vi "test-quintic-spline-05.vi"() -> ()   [LabVIEW 2019]
uses:
  <vilib>/Rock Robotics/WPI/ThirdParty/JAS_Junk/TrajLib/POSEwCURVATURE.ctl
  <vilib>/Rock Robotics/WPI/ThirdParty/JAS_Junk/TrajLib/POSE2D.ctl
  <vilib>/Rock Robotics/WPI/ThirdParty/JAS_Junk/TrajLib/TRANSLATION2D.ctl
  <vilib>/Rock Robotics/WPI/ThirdParty/JAS_Junk/TrajLib/ROTATION2D.ctl
  <vilib>/Rock Robotics/WPI/ThirdParty/JAS_Junk/TrajLib/Rotation_CreateAngle.vi
  <vilib>/Rock Robotics/WPI/ThirdParty/JAS_Junk/TrajLib/Translation_Create.vi
  <vilib>/Rock Robotics/WPI/ThirdParty/JAS_Junk/TrajLib/Util_CalcDist.vi
  <vilib>/Rock Robotics/WPI/ThirdParty/JAS_Junk/TrajLib/Trajectory_Library.lvlib
panel:
  out "XY Graph":cluster{dbl[], dbl[]}(graph)
  out "Numb\nWaypoints":i32
  out "All Interior \nwayPoints\nFound (True)":bool
  out "end rot = 0":dbl
  out "end y = 0":dbl
  out "end x = 0":dbl
  out "start rot = 0":dbl
  out "start y = 0":dbl
  out "start x = 0":dbl
  out "max dtheta < 0.0872":dbl
  out "max dy < 0.00127":dbl
  out "max dx  < 0.127":dbl
  out "Overall Error":errorcluster
  out "Elements":i32
  out "Create Spline Error":errorcluster
  out "SplinePoses\nWCurve":T1[](array[typedef]) {"POSE"."ROTATION"."SIN" format="%13.4f"; "POSE"."ROTATION"."COS" format="%13.4f"; "POSE"."ROTATION"."VALUE" format="%13.4f"; "POSE"."TRANSLATION"."Y" format="%14.3f"; "POSE"."TRANSLATION"."X" format="%14.3f"}
  out "Elapsed Time":dbl
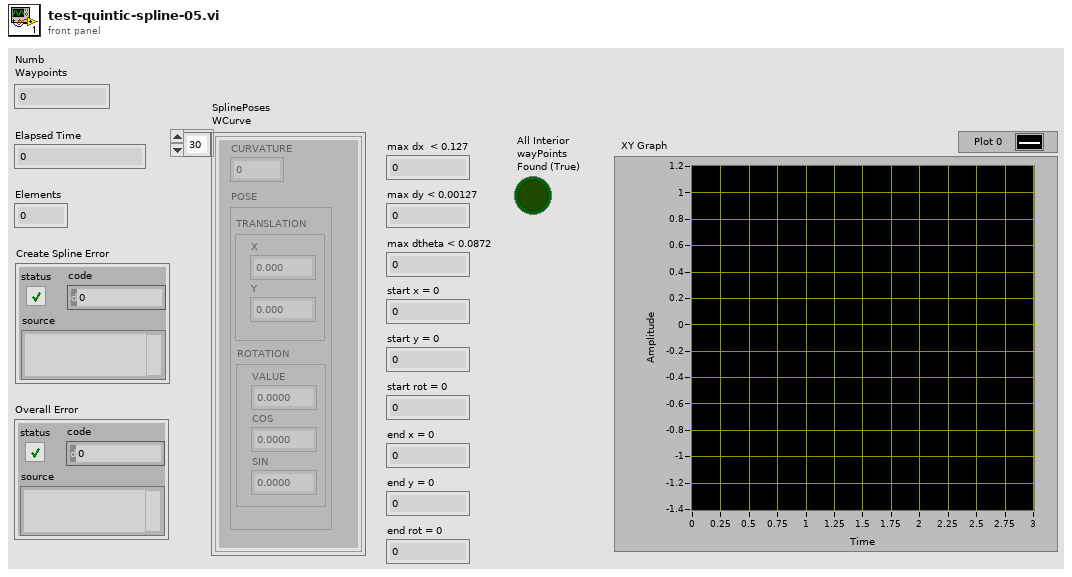
[diagram p1: front panel]
types:
  T1 = typedef "Trajectory_Library.lvlib/POSEwCURVATURE.ctl" = cluster{"CURVATURE":dbl, "POSE":T2}
  T2 = typedef "Trajectory_Library.lvlib/POSE2D.ctl" = cluster{"TRANSLATION":T3, "ROTATION":T4}
  T3 = typedef "Trajectory_Library.lvlib/TRANSLATION2D.ctl" = cluster{"X":dbl, "Y":dbl}
  T4 = typedef "Trajectory_Library.lvlib/ROTATION2D.ctl" = cluster{"VALUE":dbl, "COS":dbl, "SIN":dbl}
  T5 = typedef "Trajectory_Library.lvlib/SPLINE_CTRL_VECTOR.ctl" = cluster{"Xs":dbl[], "Ys":dbl[]}
  T6 = typedef "Trajectory_Library.lvlib/SPLINE.ctl" = cluster{"Degree":i32, "Coefficients":T7}
  T7 = typedef "NI_Matrix.lvlib/RealMatrix.ctl" = dbl[][]
  T8 = typedef "Trajectory_Library.lvlib/TWIST2D.ctl" = cluster{"dX":dbl, "dY":dbl, "dTHETA":dbl}
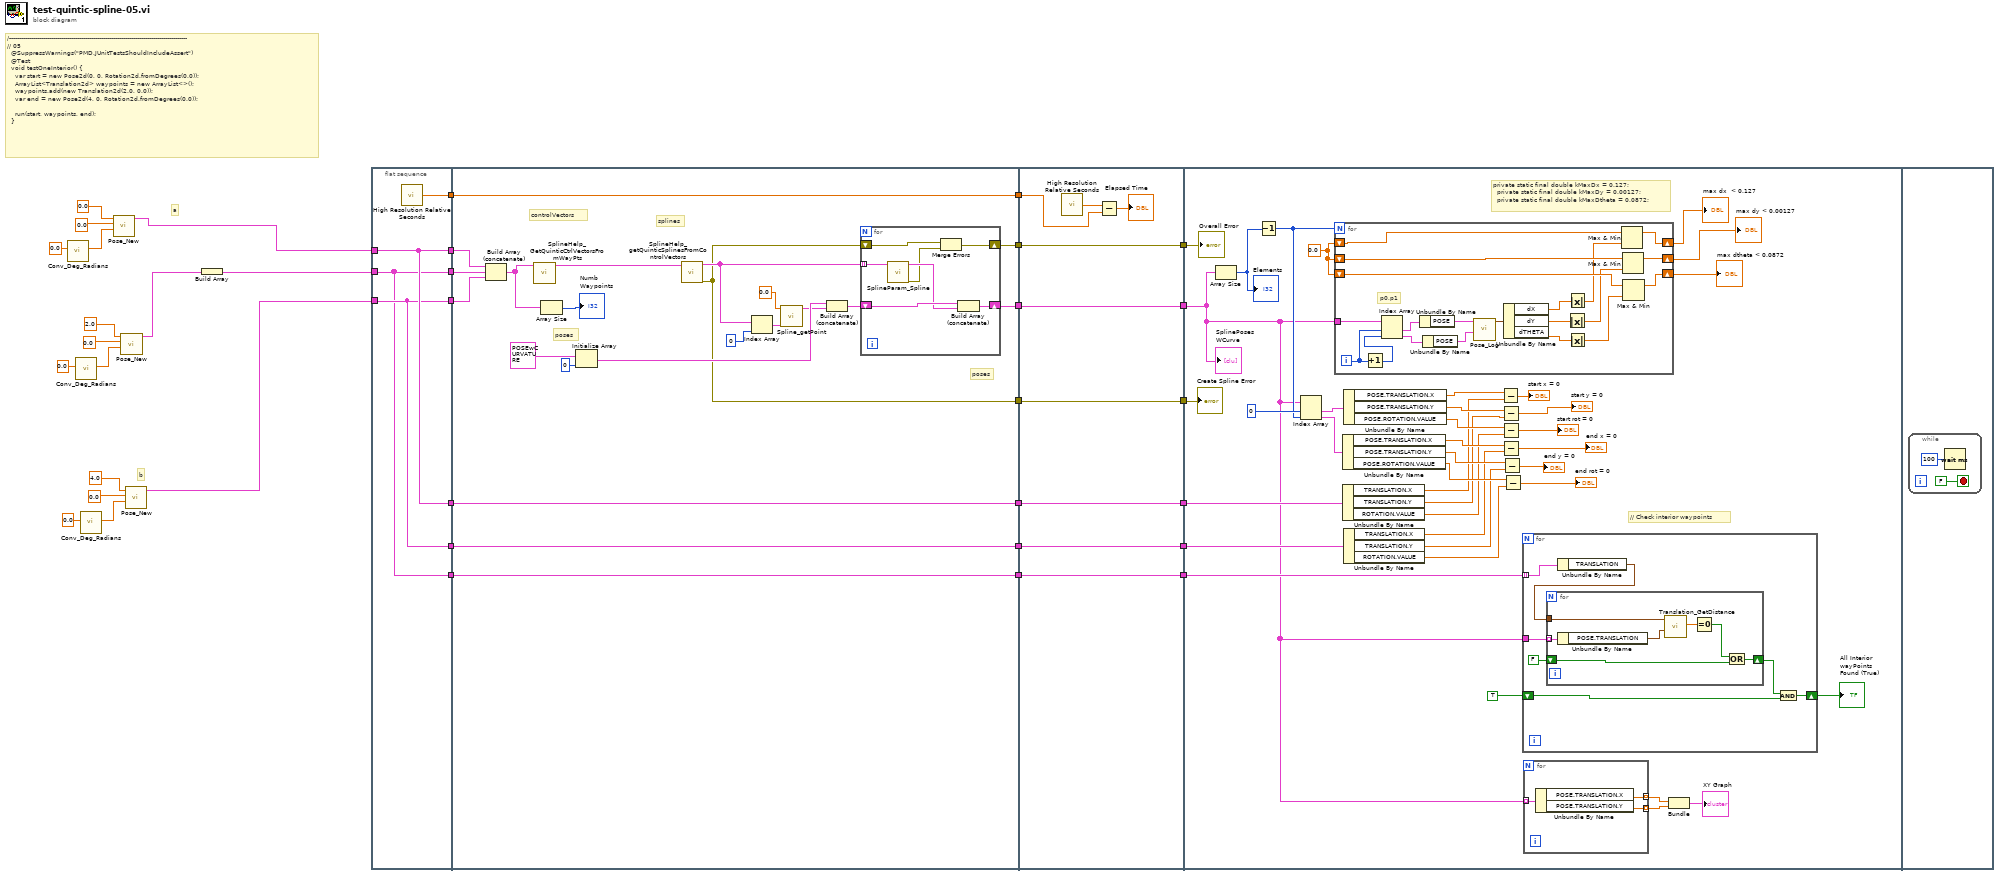
[diagram p0: block diagram]
diagram:
  # "b"
  # "a"
  # "/-----------------------------------------------------------------------------------------\n// 05\n  @SuppressWarnings(\"PMD.JUnitTestsShouldIncludeAssert\")\n  @Test\n  void testOneInterior() {\n    var start = new Pose2d(0, 0, Rotation2d.fromDegrees(0.0));\n    ArrayList<Translation2d> waypoints = new ArrayList<>();\n    waypoints.add(new Translation2d(2.0, 0.0));\n    var end = new Pose2d(4, 0, Rotation2d.fromDegrees(0.0));\n\n    run(start, waypoints, end);\n  }"
  n1 = call <vilib>:"Conv_Deg_Radians.vi"("Degress"=0.0) -> ("Radians"=w10:dbl)  [unwired: 10 in]
  n2 = call <vilib>:"Conv_Deg_Radians.vi"("Degress"=0.0) -> ("Radians"=w3:dbl)  [unwired: 10 in]
  n3 = call <vilib>:"Conv_Deg_Radians.vi"("Degress"=0.0) -> ("Radians"=w13:dbl)  [unwired: 10 in]
  n4 = call <vilib>:"Pose_New.vi"("Heading"=w10, "Y"=0.0, "X"=0.0) -> ("out POSe"=w7:T2)  [unwired: 8 in]
  n5 = call <vilib>:"Pose_New.vi"("Heading"=w3, "Y"=0.0, "X"=2.0) -> ("out POSe"=w1:T2)  [unwired: 8 in]
  n6 = call <vilib>:"Pose_New.vi"("Heading"=w13, "Y"=0.0, "X"=4.0) -> ("out POSe"=w35:T2)  [unwired: 8 in]
  n7 = Build Array(w1) -> (w6:T2[])
  n8 = flat-sequence {
    tunnel: w7 -> [w39]
    tunnel: [w39] -> w36
    tunnel: w35 -> [w38]
    tunnel: [w38] -> w34
    tunnel: [w40] -> w33
    tunnel: [w39] -> w25
    tunnel: [w38] -> w22
    tunnel: [w37] -> w17
    tunnel: w6 -> [w37]
    tunnel: [w37] -> w16
    tunnel: w36 -> [w46]
    tunnel: w34 -> [w44]
    tunnel: [w62] -> w32
    tunnel: w33 -> [w62]
    tunnel: [w52] -> w31
    tunnel: [w51] -> w29
    tunnel: [w50] -> w27
    tunnel: w25 -> [w49]
    tunnel: [w49] -> w24
    tunnel: w22 -> [w48]
    tunnel: [w48] -> w21
    tunnel: [w47] -> w18
    tunnel: w17 -> [w47]
    tunnel: w16 -> [w43]
    tunnel: w32 -> [w78]
    tunnel: w31 -> [w77]
    tunnel: [w77] -> w30
    tunnel: w29 -> [w76]
    tunnel: [w76] -> w28
    tunnel: w27 -> [w75]
    tunnel: [w75] -> w26
    tunnel: w24 -> [w72]
    tunnel: [w72] -> w23
    tunnel: w21 -> [w71]
    tunnel: [w71] -> w20
    tunnel: [w70] -> w19
    tunnel: w18 -> [w70]
    tunnel: w30 -> [w80]
    tunnel: w28 -> [w116]
    tunnel: w26 -> [w115]
    tunnel: w23 -> [w109]
    tunnel: w20 -> [w108]
    tunnel: w19 -> [w85]
    frame #0 {
      n9 = call <vilib>:"High Resolution Relative Seconds.vi"() -> ("relative seconds"=w40:dbl)
    }
    frame #1 {
      # "poses"
      # "poses"
      # "splines"
      # "controlVectors"
      n10 = Build Array (concatenate)(w46, w43, w44) -> (w42:T2[])
      n11 = call <vilib>:"SplineHelp_GetQuinticCtrlVectorsFromWayPts.vi"("WayPoints"=w42) -> ("SplineControlVectors"=w45:T5[])  [unwired: 10 in]
      n12 = Array Size(array=w42) -> (size(s)=→"Numb\nWaypoints":i32)
      n13 = Initialize Array(T1 {"CURVATURE"=0.0, "POSE"={"TRANSLATION"={"X"=0.0, "Y"=0.0}, "ROTATION"={"VALUE"=0.0, "COS"=1.0, "SIN"=0.0}}} ("POSEwCURVATURE"), 0 ("dimension size")) -> (w56:T1[])
      n14 = call <vilib>:"SplineHelp_getQuinticSplinesFromControlVectors.vi"("ControlVectors"=w45) -> ("error out"=w51:errorcluster, "splines"=w53:T6[])  [unwired: 9 in]
      n15 = Index Array(array=w53, index=0) -> (element=w58:T6)
      n16 = call <vilib>:"Spline_getPoint.vi"("inputSPLINE"=w58, "Time"=0.0) -> ("POSEwCURVATURE"=w55:T1)  [unwired: 9 in]
      n17 = Build Array (concatenate)(w56, w55) -> (w54:T1[])
      n18 = for {
        shift-right: [w66] -> w52
        shift-left: w54 -> [w68]
        tunnel: w53 -> [w69] mode=indexing
        shift-right: [w64] -> w50
        shift-left: w51 -> [w65]
        n19 = call <vilib>:"SplineParam_Spline.vi"("inputSPLINE"=w69) -> ("error out"=w63:errorcluster, "outputPOSEwCURVATURE"=w67:T1[])  [unwired: 9 in]
        n20 = Merge Errors(w65, w63) -> (w64:errorcluster)
        n21 = Build Array (concatenate)(w68, w67) -> (w66:T1[])
      }
    }
    frame #2 {
      n22 = call <vilib>:"High Resolution Relative Seconds.vi"() -> ("relative seconds"=w73:dbl)
      n23 = Subtract(x=w73, y=w78) -> (x-y=→"Elapsed Time":dbl)
    }
    frame #3 {
      w113 = 0.0
      # "// Check interior waypoints"
      # "private static final double kMaxDx = 0.127;\n  private static final double kMaxDy = 0.00127;\n  private static final double kMaxDtheta = 0.0872;"
      n24 = Array Size(array=w80) -> (size(s)=w114:i32)
      "Elements" <- w114
      n25 = Decrement(x=w114) -> (x-1=w106:i32)
      n26 = Index Array(array=w80, index #1=0 ("index"), index #2=w106) -> (element #1=w105:T1, element #2=w104:T1)
      n27 = for {
        N: w106 -> [_]
        tunnel: w80 -> [w151]
        shift-right: [w142] -> w112
        shift-left: w113 -> [w139]
        shift-right: [w140] -> w110
        shift-left: w113 -> [w137]
        shift-right: [w141] -> w111
        shift-left: w113 -> [w138]
        i -> [w153]
        # "p0,p1"
        n28 = Increment(x=w153) -> (x+1=w152:i32)
        n29 = Index Array(array=w151, index #1=w153, index #2=w152) -> (element #1=w150:T1, element #2=w149:T1)
        n30 = Unbundle By Name(w150) -> ("POSE"=w148:T2)
        n31 = Unbundle By Name(w149) -> ("POSE"=w147:T2)
        n32 = call <vilib>:"Pose_Log.vi"("end POSE"=w147, "in POSE"=w148) -> ("out TWIST"=w146:T8)  [unwired: 9 in]
        n33 = Unbundle By Name(w146) -> ("dX"=w143:dbl, "dY"=w144:dbl, "dTHETA"=w145:dbl)
        n34 = Absolute Value(x=w144) -> (abs(x)=w135:dbl)
        n35 = Absolute Value(x=w143) -> (abs(x)=w136:dbl)
        n36 = Absolute Value(x=w145) -> (abs(x)=w134:dbl)
        n37 = Max & Min(x=w139, y=w136) -> (max(x,y)=w142:dbl)  [unwired: 1 out]
        n38 = Max & Min(x=w138, y=w135) -> (max(x,y)=w141:dbl)  [unwired: 1 out]
        n39 = Max & Min(x=w137, y=w134) -> (max(x,y)=w140:dbl)  [unwired: 1 out]
      }
      "max dx  < 0.127" <- w112
      "max dy < 0.00127" <- w111
      "max dtheta < 0.0872" <- w110
      n40 = Unbundle By Name(w104) -> ("POSE.TRANSLATION.X"=w100:dbl, "POSE.TRANSLATION.Y"=w99:dbl, "POSE.ROTATION.VALUE"=w98:dbl)
      n41 = Unbundle By Name(w109) -> ("TRANSLATION.X"=w97:dbl, "TRANSLATION.Y"=w96:dbl, "ROTATION.VALUE"=w95:dbl)
      n42 = Unbundle By Name(w105) -> ("POSE.TRANSLATION.X"=w103:dbl, "POSE.TRANSLATION.Y"=w102:dbl, "POSE.ROTATION.VALUE"=w101:dbl)
      n43 = Unbundle By Name(w108) -> ("TRANSLATION.X"=w94:dbl, "TRANSLATION.Y"=w93:dbl, "ROTATION.VALUE"=w92:dbl)
      n44 = Subtract(x=w103, y=w97) -> (x-y=→"start x = 0":dbl)
      n45 = Subtract(x=w102, y=w96) -> (x-y=→"start y = 0":dbl)
      n46 = Subtract(x=w101, y=w95) -> (x-y=→"start rot = 0":dbl)
      n47 = Subtract(x=w100, y=w94) -> (x-y=→"end x = 0":dbl)
      n48 = Subtract(x=w99, y=w93) -> (x-y=→"end y = 0":dbl)
      n49 = Subtract(x=w98, y=w92) -> (x-y=→"end rot = 0":dbl)
      n50 = for {
        tunnel: w85 -> [w121] mode=indexing
        tunnel: w80 -> [w126]
        shift-right: [w125] -> w83
        shift-left: TRUE -> [w124]
        n51 = Unbundle By Name(w121) -> ("TRANSLATION"=w120:T3)
        n52 = for {
          tunnel: w126 -> [w130] mode=indexing
          shift-right: [w133] -> w122
          shift-left: FALSE -> [w132]
          tunnel: w120 -> [w131]
          n53 = Unbundle By Name(w130) -> ("POSE.TRANSLATION"=w129:T3)
          n54 = call <vilib>:"Translation_GetDistance.vi"("other Translation"=w129, "In Translation"=w131) -> ("Distance"=w128:dbl)  [unwired: 9 in]
          n55 = Equal To 0?(x=w128) -> (x = 0?=w127:bool)
          n56 = Or(x=w127, y=w132) -> (x .or. y?=w133:bool)
        }
        n57 = And(x=w122, y=w124) -> (x .and. y?=w125:bool)
      }
      "All Interior \nwayPoints\nFound (True)" <- w83
      n58 = for {
        tunnel: [w119] -> w82 mode=indexing
        tunnel: [w118] -> w81 mode=indexing
        tunnel: w80 -> [w117] mode=indexing
        n59 = Unbundle By Name(w117) -> ("POSE.TRANSLATION.X"=w119:dbl, "POSE.TRANSLATION.Y"=w118:dbl)
      }
      n60 = Bundle(w82, w81) -> (→"XY Graph":cluster{dbl[], dbl[]})  [unwired: 1 in]
      "SplinePoses\nWCurve" <- w80
      "Create Spline Error" <- w116
      "Overall Error" <- w115
    }
    frame #4 {
      n61 = while {
        stop <- FALSE stop-if-true
        n62 = Wait (ms)(milliseconds to wait=u32 100) -> ()  [unwired: 1 out]
      }
    }
  }
